vi "AnalogDemultiplex_AND_FIXED_samples_3GHz.vi"(0 "Analog data cluster":T1, 5 "Over? Array":bool[](array[boolean])=[FALSE, FALSE, FALSE, FALSE, FALSE, FALSE, FALSE, FALSE], 7 "Last Sample A1":u8, 9 "Last Sample A2":u8, 11 "Last? Input":bool, 12 "array in":bool[](array[boolean])=[FALSE, FALSE, FALSE, FALSE, FALSE, FALSE, FALSE, FALSE, FALSE, FALSE, FALSE, FALSE, FALSE]) -> (4 "Data A1 out":u64, 6 "Data A2 out":u64, 14 "array out":bool[](array[boolean]), 15 "Last? Output":bool)   [LabVIEW 2014]
panel:
  out "Wrap Output":bool
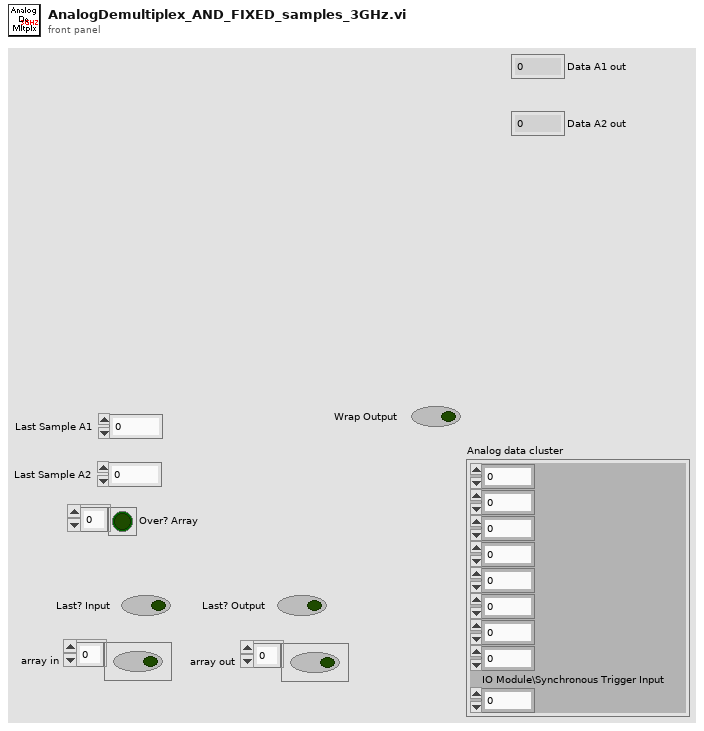
[diagram p1: front panel]
types:
  T1 = cluster{u16, u16, u16, u16, u16, u16, u16, u16, "IO Module\\Synchronous Trigger Input":u8}
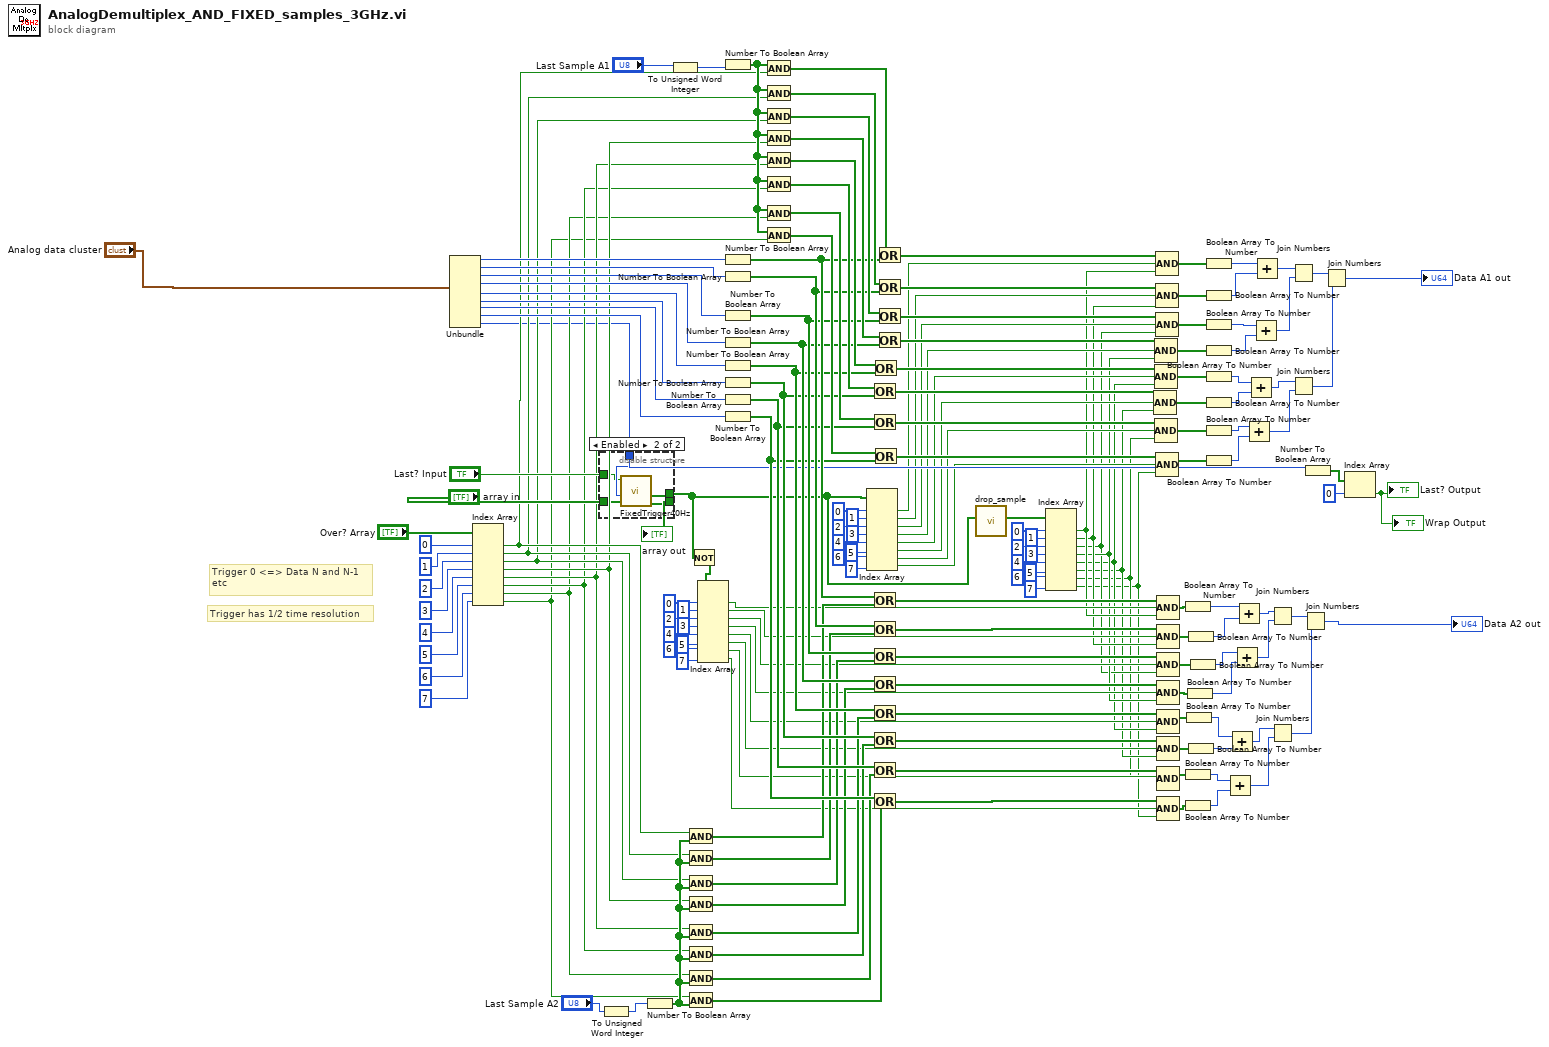
[diagram p0: block diagram]
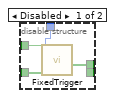
[diagram p2: hidden frame]
diagram:
  # "Trigger 0 <=> Data N and N-1\netc"
  # "Trigger has 1/2 time resolution"
  n1 = Unbundle("Analog data cluster") -> (w159:u16, w158:u16, w157:u16, w156:u16, w155:u16, w154:u16, w153:u16, w152:u16, "IO Module\\Synchronous Trigger Input"=w78:u8)
  n2 = Index Array(array="Over? Array", index #1=0 ("index"), index #2=1 ("index"), index #3=2 ("index"), index #4=3 ("index"), index #5=4 ("index"), index #6=5 ("index"), index #7=6 ("index"), index #8=7 ("index")) -> (element #1=w128:bool, element #2=w127:bool, element #3=w126:bool, element #4=w125:bool, element #5=w124:bool, element #6=w123:bool, element #7=w122:bool, element #8=w121:bool)
  n3 = disable-structure shown="Enabled" {
    disable-tunnel: "Last? Input" -> [w180 w183]
    disable-tunnel: "array in" -> [w177 w184]
    disable-tunnel: [_ w181] -> w172
    disable-tunnel: w78 -> [w179 w185]
    disable-tunnel: [w178 w182] -> w47
    frame Disabled {
      n4 = call "FixedTrigger.vi"("array in"=w177, "IO Module\\Synchronous Trigger Input"=w179, "Last? Input"=w180) -> ("trigger out"=w178:bool[])  [unwired: 7 in, 1 out]
    }
    frame Enabled {
      n5 = call "FixedTrigger40Hz.vi"("array in"=w184, "IO Module\\Synchronous Trigger Input"=w185, "Last? Input"=w183) -> ("array out"=w181:bool[], "trigger out"=w182:bool[])  [unwired: 7 in]
    }
  }
  "array out" <- w172
  n6 = To Unsigned Word Integer(number="Last Sample A2") -> (unsigned 16bit integer=w3:u16)
  n7 = Number To Boolean Array(number=w3) -> (Boolean array=w129:bool[])
  n8 = To Unsigned Word Integer(number="Last Sample A1") -> (unsigned 16bit integer=w1:u16)
  n9 = And(x=w128, y=w129) -> (x .and. y?=w88:bool[])
  n10 = And(x=w127, y=w129) -> (x .and. y?=w87:bool[])
  n11 = And(x=w126, y=w129) -> (x .and. y?=w86:bool[])
  n12 = And(x=w125, y=w129) -> (x .and. y?=w85:bool[])
  n13 = And(x=w124, y=w129) -> (x .and. y?=w81:bool[])
  n14 = And(x=w123, y=w129) -> (x .and. y?=w82:bool[])
  n15 = And(x=w122, y=w129) -> (x .and. y?=w83:bool[])
  n16 = And(x=w121, y=w129) -> (x .and. y?=w84:bool[])
  n17 = Not(x=w47) -> (.not. x?=w73:bool[])
  n18 = Index Array(array=w73, index #1=0 ("index"), index #2=1 ("index"), index #3=2 ("index"), index #4=3 ("index"), index #5=4 ("index"), index #6=5 ("index"), index #7=6 ("index"), index #8=7 ("index")) -> (element #1=w72:bool, element #2=w71:bool, element #3=w70:bool, element #4=w69:bool, element #5=w68:bool, element #6=w67:bool, element #7=w66:bool, element #8=w65:bool)
  n19 = Number To Boolean Array(number=w1) -> (Boolean array=w130:bool[])
  n20 = Number To Boolean Array(number=w159) -> (Boolean array=w104:bool[])
  n21 = Number To Boolean Array(number=w158) -> (Boolean array=w103:bool[])
  n22 = Number To Boolean Array(number=w157) -> (Boolean array=w102:bool[])
  n23 = Number To Boolean Array(number=w156) -> (Boolean array=w101:bool[])
  n24 = Number To Boolean Array(number=w155) -> (Boolean array=w100:bool[])
  n25 = Number To Boolean Array(number=w154) -> (Boolean array=w99:bool[])
  n26 = Number To Boolean Array(number=w153) -> (Boolean array=w98:bool[])
  n27 = Number To Boolean Array(number=w152) -> (Boolean array=w97:bool[])
  n28 = And(x=w130, y=w128) -> (x .and. y?=w105:bool[])
  n29 = And(x=w130, y=w127) -> (x .and. y?=w106:bool[])
  n30 = And(x=w130, y=w126) -> (x .and. y?=w107:bool[])
  n31 = And(x=w130, y=w125) -> (x .and. y?=w108:bool[])
  n32 = And(x=w130, y=w124) -> (x .and. y?=w109:bool[])
  n33 = And(x=w130, y=w123) -> (x .and. y?=w110:bool[])
  n34 = And(x=w130, y=w122) -> (x .and. y?=w111:bool[])
  n35 = And(x=w130, y=w121) -> (x .and. y?=w112:bool[])
  n36 = Index Array(array=w47, index #1=0 ("index"), index #2=1 ("index"), index #3=2 ("index"), index #4=3 ("index"), index #5=4 ("index"), index #6=5 ("index"), index #7=6 ("index"), index #8=7 ("index")) -> (element #1=w55:bool, element #2=w54:bool, element #3=w53:bool, element #4=w52:bool, element #5=w51:bool, element #6=w50:bool, element #7=w49:bool, element #8=w48:bool)
  n37 = Or(x=w110, y=w99) -> (x .or. y?=w118:bool[])
  n38 = Or(x=w111, y=w98) -> (x .or. y?=w119:bool[])
  n39 = Or(x=w104, y=w88) -> (x .or. y?=w96:bool[])
  n40 = Or(x=w103, y=w87) -> (x .or. y?=w95:bool[])
  n41 = Or(x=w102, y=w86) -> (x .or. y?=w94:bool[])
  n42 = Or(x=w101, y=w85) -> (x .or. y?=w93:bool[])
  n43 = Or(x=w100, y=w81) -> (x .or. y?=w92:bool[])
  n44 = Or(x=w99, y=w82) -> (x .or. y?=w91:bool[])
  n45 = Or(x=w98, y=w83) -> (x .or. y?=w90:bool[])
  n46 = Or(x=w97, y=w84) -> (x .or. y?=w89:bool[])
  n47 = Or(x=w109, y=w100) -> (x .or. y?=w117:bool[])
  n48 = Or(x=w112, y=w97) -> (x .or. y?=w120:bool[])
  n49 = Or(x=w105, y=w104) -> (x .or. y?=w113:bool[])
  n50 = Or(x=w106, y=w103) -> (x .or. y?=w114:bool[])
  n51 = Or(x=w107, y=w102) -> (x .or. y?=w115:bool[])
  n52 = Or(x=w108, y=w101) -> (x .or. y?=w116:bool[])
  n53 = call "drop_sample.vi"("trigger in"=w47) -> ("drop sample"=w38:bool[])  [unwired: 10 in]
  n54 = Index Array(array=w38, index #1=0 ("index"), index #2=1 ("index"), index #3=2 ("index"), index #4=3 ("index"), index #5=4 ("index"), index #6=5 ("index"), index #7=6 ("index"), index #8=7 ("index")) -> (element #1=w37:bool, element #2=w36:bool, element #3=w34:bool, element #4=w35:bool, element #5=w33:bool, element #6=w32:bool, element #7=w31:bool, element #8=w30:bool)
  n55 = Compound Arithmetic op=AND(w118, w50, w32) -> (w141:bool[])
  n56 = Compound Arithmetic op=AND(w116, w52, w35) -> (w140:bool[])
  n57 = Compound Arithmetic op=AND(w117, w51, w33) -> (w164:bool[])
  n58 = Compound Arithmetic op=AND(w119, w49, w31) -> (w165:bool[])
  n59 = Compound Arithmetic op=AND(w113, w55, w37) -> (w162:bool[])
  n60 = Compound Arithmetic op=AND(w114, w54, w36) -> (w147:bool[])
  n61 = Compound Arithmetic op=AND(w115, w53, w34) -> (w163:bool[])
  n62 = Compound Arithmetic op=AND(w120, w48, w30) -> (w142:bool[])
  n63 = Compound Arithmetic op=AND(w96, w72, w37) -> (w168:bool[])
  n64 = Compound Arithmetic op=AND(w95, w71, w36) -> (w143:bool[])
  n65 = Compound Arithmetic op=AND(w94, w70, w34) -> (w169:bool[])
  n66 = Compound Arithmetic op=AND(w93, w69, w35) -> (w144:bool[])
  n67 = Compound Arithmetic op=AND(w92, w68, w33) -> (w170:bool[])
  n68 = Compound Arithmetic op=AND(w91, w67, w32) -> (w145:bool[])
  n69 = Compound Arithmetic op=AND(w90, w66, w31) -> (w171:bool[])
  n70 = Compound Arithmetic op=AND(w89, w65, w30) -> (w146:bool[])
  n71 = Boolean Array To Number(Boolean array=w168) -> (number=w28:u16)
  n72 = Boolean Array To Number(Boolean array=w171) -> (number=w20:u16)
  n73 = Boolean Array To Number(Boolean array=w146) -> (number=w19:u16)
  n74 = Boolean Array To Number(Boolean array=w170) -> (number=w22:u16)
  n75 = Boolean Array To Number(Boolean array=w144) -> (number=w24:u16)
  n76 = Boolean Array To Number(Boolean array=w143) -> (number=w27:u16)
  n77 = Boolean Array To Number(Boolean array=w145) -> (number=w21:u16)
  n78 = Boolean Array To Number(Boolean array=w169) -> (number=w25:u16)
  n79 = Boolean Array To Number(Boolean array=w162) -> (number=w16:u16)
  n80 = Boolean Array To Number(Boolean array=w147) -> (number=w15:u16)
  n81 = Boolean Array To Number(Boolean array=w163) -> (number=w14:u16)
  n82 = Boolean Array To Number(Boolean array=w140) -> (number=w13:u16)
  n83 = Boolean Array To Number(Boolean array=w164) -> (number=w12:u16)
  n84 = Boolean Array To Number(Boolean array=w141) -> (number=w11:u16)
  n85 = Boolean Array To Number(Boolean array=w165) -> (number=w10:u16)
  n86 = Boolean Array To Number(Boolean array=w142) -> (number=w9:u16)
  n87 = Add(x=w20, y=w19) -> (x+y=w18:u16)
  n88 = Add(x=w22, y=w21) -> (x+y=w17:u16)
  n89 = Add(x=w25, y=w24) -> (x+y=w23:u16)
  n90 = Add(x=w28, y=w27) -> (x+y=w26:u16)
  n91 = Add(x=w10, y=w9) -> (x+y=w8:u16)
  n92 = Add(x=w12, y=w11) -> (x+y=w7:u16)
  n93 = Add(x=w14, y=w13) -> (x+y=w6:u16)
  n94 = Add(x=w16, y=w15) -> (x+y=w5:u16)
  n95 = Join Numbers(hi=w26, lo=w23) -> ((hi.lo)=w167:u32)
  n96 = Join Numbers(hi=w17, lo=w18) -> ((hi.lo)=w166:u32)
  n97 = Join Numbers(hi=w5, lo=w6) -> ((hi.lo)=w161:u32)
  n98 = Join Numbers(hi=w7, lo=w8) -> ((hi.lo)=w160:u32)
  n99 = Join Numbers(hi=w167, lo=w166) -> ((hi.lo)=→"Data A2 out":u64)
  n100 = Number To Boolean Array(number=w78) -> (Boolean array=w79:bool[])
  n101 = Join Numbers(hi=w161, lo=w160) -> ((hi.lo)=→"Data A1 out":u64)
  n102 = Index Array(array=w79, index=0) -> (element=→"Last? Output" →"Wrap Output":bool)
